vi "VI Under Test.vi"(10 "N2":dbl=2.0, 11 "N1":dbl=1.0) -> (3 "Result":dbl=3.0)   [LabVIEW 2023]
doc: "Demonstrates how to use a user-defined comparison VI in the LabVIEW Unit Test Framework Toolkit. Use this VI as a VI under test in this example."
panel:
  # "Overview: Demonstrates how to use a user-defined comparison VI in the LabVIEW Unit Test Framework Toolkit.\nRequirements: LabVIEW Full Development System, Unit Test Framework Toolkit\nInstructions: \n1.  Execute the VI under Test_Pass.lvtest test file for this VI.\n     a) \tIn the Project Explorer window, expand the Unit Test Files folder, right-click VI under Test_Pass.lvtest, and select Run \n          from the shortcut menu. \n     b)\t View the test results in the Unit Test Framework Results window, which shows that this test passes.\n           In the Project Explorer window, double-click VI under Test_Pass.lvtest to display the Test Properties dialog box. Read\n           the comment on the Configuration page to understand why this test passes.\n2.\t Execute the VI under Test_Fail.lvtest test file for this VI.\n     a) \tIn the Project Explorer window, right-click VI under Test_Fail.lvtest and select Run from the shortcut menu.\n     b) \tView the test results in the Unit Test Framework Results window, which shows that this test passes.\n     c) \tIn the Project Explorer window, double-click VI under Test_Pass.lvtest to display the Test Properties dialog box. Read \n          the comment on the Configuration page to understand why this test fails."
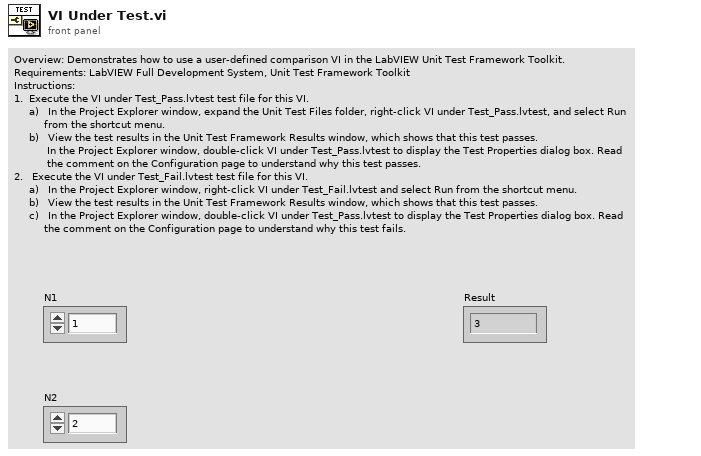
[diagram p1: front panel]
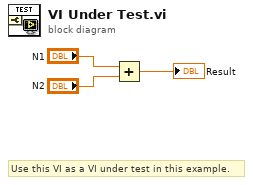
[diagram p0: block diagram]
diagram:
  # "Use this VI as a VI under test in this example."
  n1 = Add(x="N1", y="N2") -> (x+y=→"Result":dbl)
